vi "wymiennik ciepla z recyklem.vi"() -> ()   [LabVIEW 2013]
uses:
  <vilib>/Utility/file.llb/Write To Spreadsheet File (DBL).vi
panel:
  in  "Time STOP":bool=TRUE
  out "Tex deg.C":dbl=5.0
  out "F l/min":dbl=3.6999999999999997
  in  "Enable temperature profiles":bool=TRUE
  out "?":dbl[][](graph)=[[79.48766614690592, 79.44291247956771, 79.39728659693863, 79.35077150019917, 79.30334985923562, 79.25500400618341, 79.20571592884455, 79.15546726397692, 79.1042392904526, 79.05201292228297, 78.99876870150788, 78.94448679094619, 78.889146966805, 78.83272861114493, 78.77521070419847, 78.71657181653867, 78.6567901010952, 78.59584328501471, 78.53370866136277, 78.47036308066384, 78.40578294227656, 78.33994418560081, 78.27282228111352, 78.20439222122963, 78.1346285109851, 78.06350515853822, 77.99099566548585, 77.91707301699094, 77.84170967171757, 77.76487755156991, 77.68654803123121, 77.60669192749882, 77.52527948841141, 77.44228038216438, 77.35766368580904, 77.27139787373171, 77.18345080590827, 77.09378971592965, 77.00238119879418, 76.90919119846187, 76.81418499516609, 76.71732719247811, 76.61858170411948, 76.51791174051729, 76.41527979509759, 76.31064763031151, 76.20397626338914, 76.09522595181573, 75.98435617852483, 75.87132563680287, 75.75609221489948, 75.63861298033804, 75.51884416392022, 75.39674114341899, 75.2722584269537, 75.14534963604116, 75.01596748831648, 74.88406377991706, 74.7495893675233, 74.61249415004929, 74.47272704997664, 74.33023599432462, 74.18496789524929, 74.03686863026455, 73.88588302207783, 73.73195481803263, 73.57502666915053, 73.41504010876469, 73.2519355307369, 73.08565216725025, 72.91612806616875, 72.74330006795597, 72.56710378214362, 72.38747356334164, 72.20434248678075, 72.01764232337828, 71.8273035143181, 71.63325514513511, 71.43542491929466, 71.23373913125705, 71.0281226390171, 70.81849883610849, 70.60478962306254, 70.38691537831073, 70.16479492852007, 69.93834551835042, 69.70748277962235, 69.47212069988414, 69.23217159036608, 68.98754605331037, 68.7381529486642, 68.4838993601237, 68.22469056051622, 67.9604299765078, 67.69101915262286, 67.41635771456275, 67.13634333180926, 66.85087167949942, 66.5598363995572, 66.26312906106772, 65.96063911987918], [71.36651285431357, 71.1634840219988, 70.95649831055961, 70.74547860340017, 70.53034628098024, 70.31102119152389, 70.08742162115745, 69.8594642634653, 69.62706418845255, 69.39013481090258, 69.1485878581181, 68.9023333370334, 68.65127950068562, 68.39533281403267, 68.1343979191049, 67.8683775994776, 67.59717274405111, 67.32068231012504, 67.03880328575283, 66.75143065136263, 66.45845734063013, 66.15977420058901, 65.85526995096376, 65.54483114271005, 65.2283421157471, 64.90568495586618, 64.57673945079941, 64.24138304543229, 63.89949079614336, 63.55093532425402, 63.19558676857114, 62.833312737004654, 62.46397825724232, 62.08744572646311, 61.703574860070596, 61.312222639427155, 60.91324325856956, 60.50648806988611, 60.09180552873504, 59.66904113698357, 59.23803738544663, 58.79863369520366, 58.35066635777182, 57.893968474113144, 57.428369892453055, 56.95369714488696, 56.46977338275136, 55.97641831073543, 55.47344811970844, 54.960675418238054, 54.43790916277395, 53.90495458647083, 53.361613126624164, 52.80768235069178, 52.242955880873616, 51.667223317221634, 51.080270159251164, 50.48187772602455, 49.87182307467725, 49.24987891735612, 48.61581353653881, 47.96939069870288, 47.31036956631235, 46.638504608088944, 45.95354550753457, 45.255237069671004, 44.54331912596198, 43.817526437382284, 43.07758859559774, 42.32322992221928, 41.55416936609352, 40.77012039859166, 39.970790906857566, 39.15588308497543, 38.32509332301629, 37.4781120939222, 36.614623838185814, 35.73430684628252, 34.83683313881122, 33.921868344299156, 32.98907157462523, 32.03809529801545, 31.06858520956314, 30.08018009922566, 29.072511717248542, 28.045204636966762, 26.99787611493218, 25.930135948314934, 24.84158632952571, 23.73182169800471, 22.600428589122075, 21.44698548013353, 20.271062633133784, 19.07222193494923, 17.850016733910273, 16.603991673442465, 15.333682522414465, 14.038616002179598, 12.718309610246605, 11.372271440513844, 10.0]]
  in  "Ph":dbl(knob)=1.0 caption="C %" min=0.0 max=1.0 step=0.001 scale=0.0..1.0
  in  "Automation mode":u8(knob)=2 caption="C %" scale=0.0..2.0
  out "Ph":dbl(knob)=1.0 scale=0.0..1.0
  out "F l/min":dbl(knob)=3.6999999999999997 scale=0.0..5.0
  out "Fc l/min":dbl(knob)=0.7999999999999993 scale=0.0..5.0
  in  "?":bool
  in  "?":bool
  out "Txou deg. C":dbl=65.96063911987918
  out "Txin deg.C":dbl=79.48766614690592
  out "Tcou deg.C":dbl=71.36651285431357
  out "Fc l/min":dbl=0.7999999999999993
  out "Tcin deg.C":dbl=10.0
  in  "Auto":bool
  in  "Scaled RT interval":dbl min=0.001 max=2.0 step=0.001 format="%.3f"
  in  "NIS":dbl=600.0 min=0.0 step=1.0
  in  "Dt":dbl=1.0 min=0.0 step=1.0
  out "t  min\nmin]":dbl=2484.1883333711858
  in  "Tab Control":enum32{"Parameters ", "Manual", "Auto"}(tab)
  in  "Vh [l]":dbl=0.25 min=0.0 step=0.01 format="%.2f"
  in  "Vc [l]":dbl=0.8 min=0.0 step=0.1 format="%.1f"
  in  "Vx [l]":dbl=0.8 min=0.0 step=0.1 format="%.1f"
  in  "n":u32=100 min=2 step=1
  in  "hc[l/min]":dbl=2.0 min=0.0 step=1.0 format="%.2f"
  in  "hx[l/min]":dbl=2.0 min=0.0 step=1.0 format="%.2f"
  in  "ah [deg.C*l/min]":dbl=50.05 min=0.0 step=1.0 format="%.1f"
  in  "bc [l/min]":dbl min=0.0 step=0.05 format="%.2f"
  in  "bx[l/min]":dbl min=0.0 step=0.05 format="%.2f"
  in  "bh[l/min]":dbl min=0.0 step=0.05 format="%.2f"
  in  "Tcin [deg.C]":dbl=10.0 min=0.0 step=1.0
  in  "Fc [l/min]":dbl=0.7999999999999993 min=0.0 step=0.1 format="%.1f"
  in  "F [l/min]":dbl=3.6999999999999997 min=0.0 step=0.1 format="%.1f"
  in  "Thin [deg.C]":dbl=10.0 min=0.0 step=1.0
  in  "Tex[deg.C]":dbl=5.0 min=0.0 step=1.0
  in  "Fcmax [l/min]":dbl=4.0 min=0.0 step=0.1 format="%.1f"
  in  "Fmax [l/min]":dbl=4.0 min=0.0 step=0.1 format="%.1f"
  in  "Fcmin [l/min]":dbl=0.8 min=0.0 step=0.1 format="%.1f"
  in  "Steady state [min]":dbl=10.0 min=0.0 step=1.0
  in  "N2":dbl=10.0 min=0.0 step=1.0
  in  "Phmin":dbl=0.5 min=0.0 step=0.1 format="%.1f"
  in  "Fmin [l/min]":dbl=0.8 min=0.0 step=0.1 format="%.1f"
  in  "Phmax":dbl=1.0 min=0.0 max=1.0 step=0.1 format="%.1f"
  in  "N1":dbl=10.0 min=0.0 step=1.0
  out "Time charts":T1(graph)={"Tkoncowa"=71.36651285431357, "F2auto"=79.48766614690592, 65.96063911987918, "F1auto"=3.6999999999999997, "Twy"=0.7999999999999993, "Twe"=1.0}
  # "Tcou"
  # "80"
  # "deg.C"
  # "10"
  # "Txin/Thou"
  # "90"
  # "deg.C"
  # "10"
  # "Txou/Thin"
  # "50"
  # "deg.C"
  # "10"
  # "F"
  # "5"
  # "l/min"
  # "0"
  # "Fc"
  # "5"
  # "l/min"
  # "Manual"
  # "0"
  # "Ph"
  # "1"
  # "0"
  # "Fc"
  # "F"
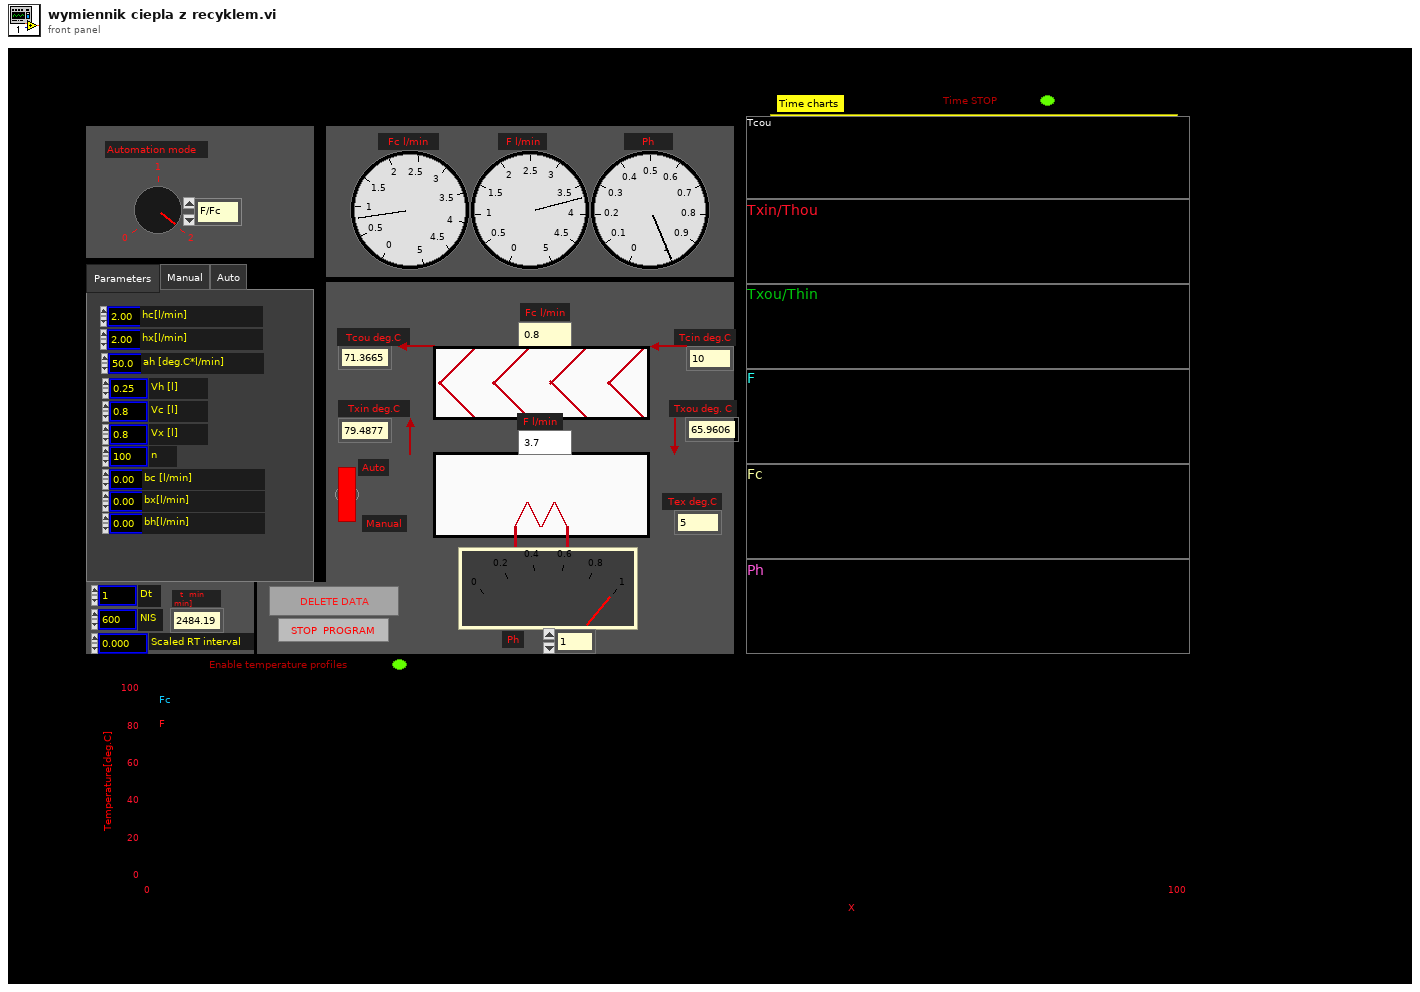
[diagram p1: front panel]
types:
  T1 = cluster{"Tkoncowa":dbl, "F2auto":dbl, dbl, "F1auto":dbl, "Twy":dbl, "Twe":dbl}
  T2 = cluster{"Tkoncowa":dbl, "Twy":dbl, "Twe":dbl, dbl, dbl, dbl}
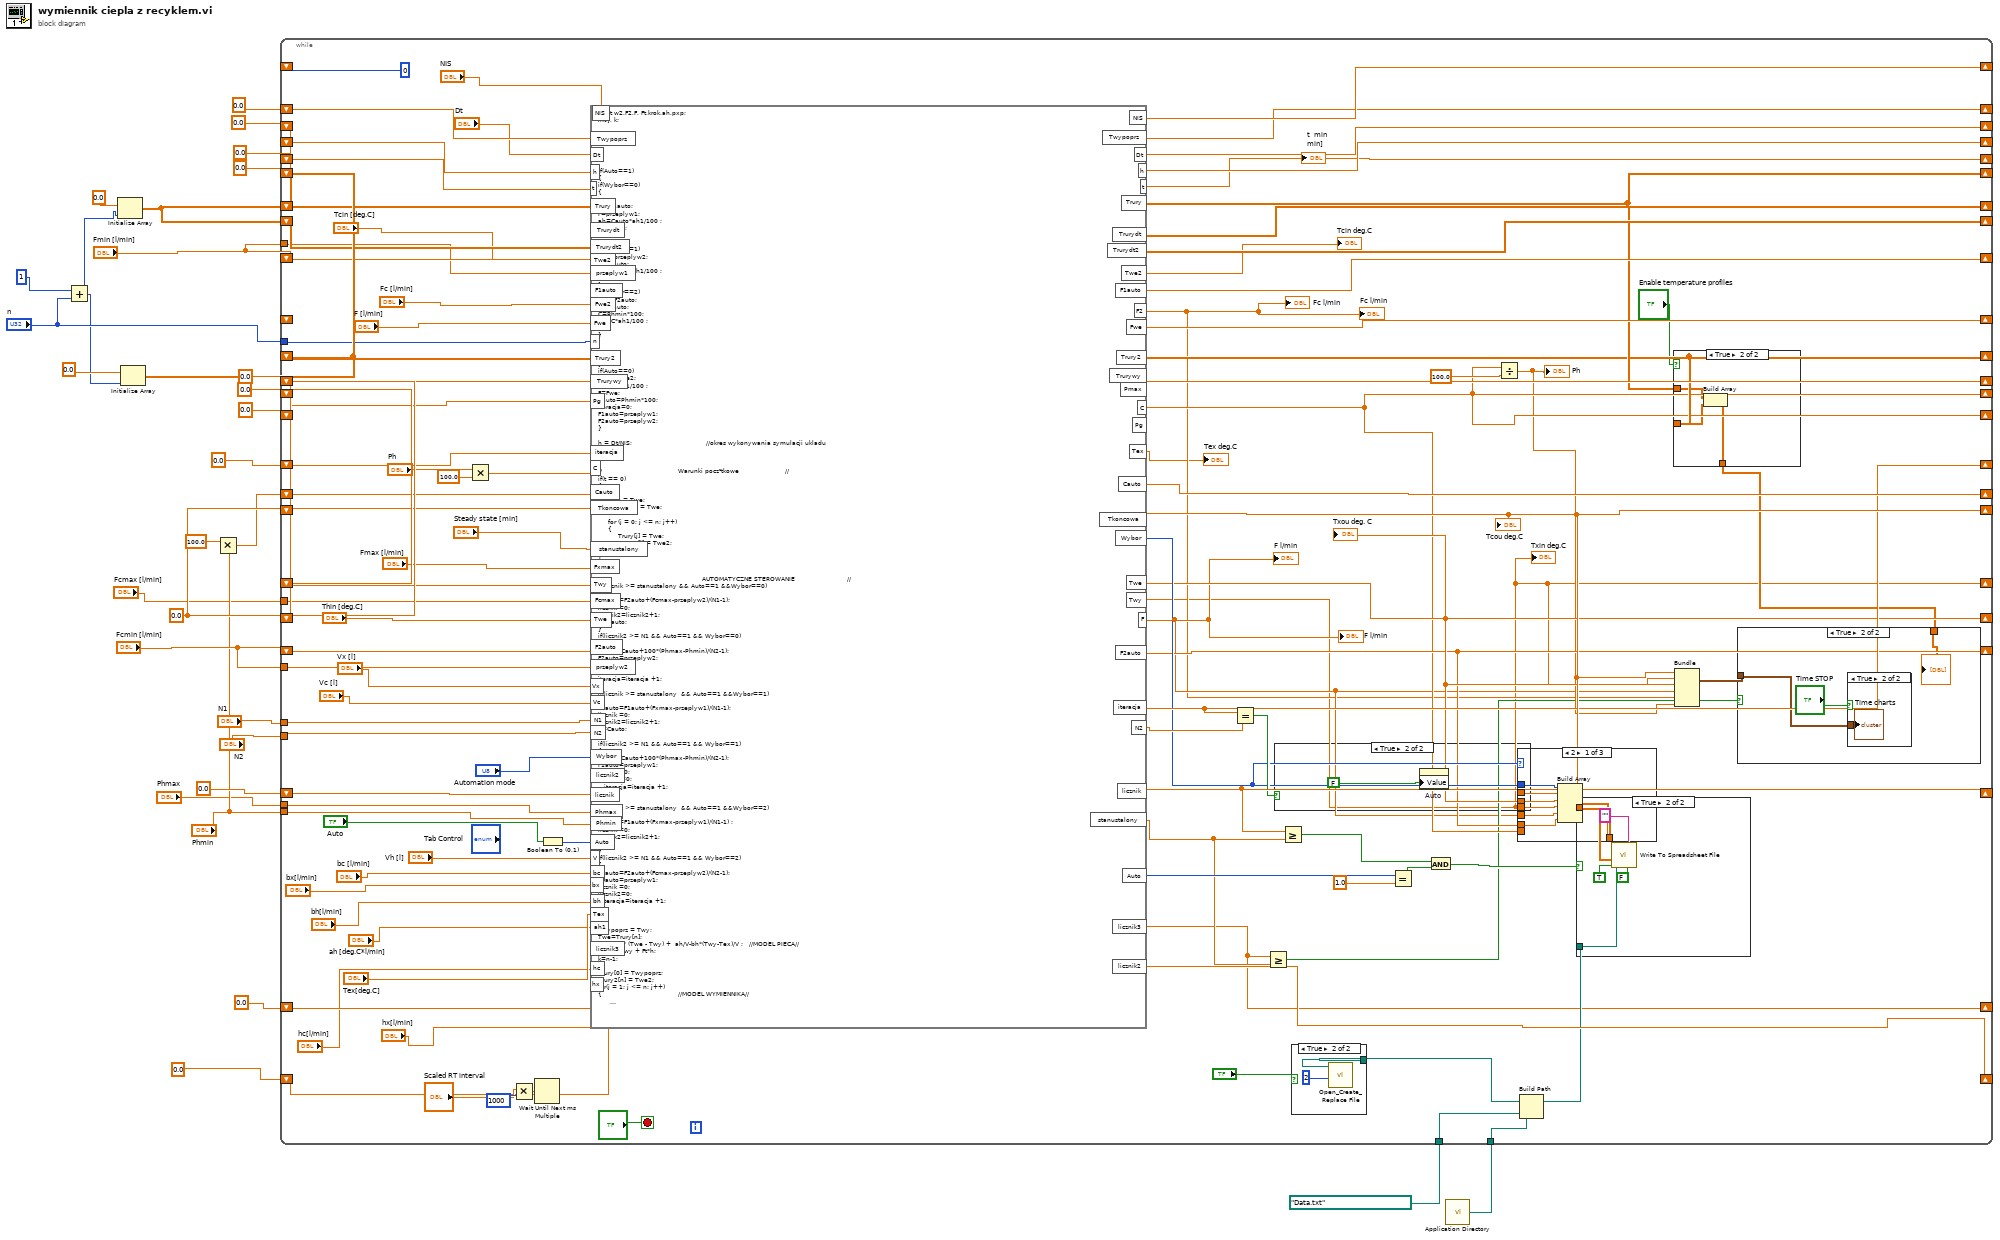
[diagram p0: block diagram]
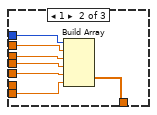
[diagram p5: hidden frame]
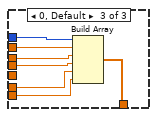
[diagram p6: hidden frame]
diagram:
  w19 = 0.0
  n1 = Add(x=1, y="n") -> (x+y=w2:u32)
  n2 = Initialize Array "Initialize Array"(0.0, w2) -> (w21:dbl[])
  n3 = Initialize Array "Initialize Array"(0.0, w2) -> (w22:dbl[])
  n4 = Multiply(x=100.0, y="Phmin") -> (x*y=w9:dbl)
  n5 = call <vilib>:"Application Directory.vi"() -> ("Application Directory"=w16:path)
  n6 = while {
    shift-right: [w106] -> _
    shift-left: 0.0 -> [w115]
    shift-right: [w32] -> _
    shift-left: 0.0 -> [w131]
    shift-right: [w110] -> _
    shift-left: 0.0 -> [w130]
    shift-right: [w122] -> _
    shift-left: 0.0 -> [w129]
    shift-right: [w52] -> _
    shift-left: _ -> [_]
    shift-right: [w77] -> _
    shift-left: 0.0 -> [_]
    shift-right: [w60] -> _
    shift-left: w22 -> [w128]
    shift-right: [w120] -> _
    shift-left: w21 -> [w119]
    shift-right: [w89] -> _
    shift-left: w19 -> [w127]
    shift-right: [w121] -> _
    shift-left: 0 -> [_]
    shift-right: [w123] -> _
    shift-left: 0.0 -> [_]
    shift-right: [w59] -> _
    shift-left: w22 -> [w118]
    shift-right: [w116] -> _
    shift-left: w21 -> [w117]
    shift-right: [w114] -> _
    shift-left: _ -> [_]
    shift-right: [w75] -> _
    shift-left: "Fcmin [l/min]" -> [w113]
    shift-right: [w111] -> _
    shift-left: 0.0 ("licznik") -> [w112]
    shift-right: [w88] -> _
    shift-left: 0.0 ("licznik") -> [w57]
    shift-right: [w86] -> _
    shift-left: w19 -> [w109]
    shift-right: [w87] -> _
    shift-left: w9 -> [w101]
    shift-right: [w52] -> _
    shift-left: 0.0 -> [w100]
    shift-right: [w76] -> _
    shift-left: "Fmin [l/min]" -> [w99]
    tunnel: "Fcmin [l/min]" -> [w97]
    tunnel: "Fmin [l/min]" -> [w96]
    shift-right: [w84] -> _
    shift-left: 0.0 ("licznik") -> [w92]
    tunnel: w16 -> [w91]
    tunnel: path "Data.txt" -> [w90]
    tunnel: "N1" -> [w83]
    tunnel: "N2" -> [w82]
    tunnel: "Phmin" -> [w64]
    tunnel: "Fcmax [l/min]" -> [w63]
    tunnel: "Phmax" -> [w62]
    tunnel: "n" -> [w61]
    shift-right: [w46] -> _
    shift-left: 0.0 ("licznik") -> [w47]
    stop <- "?" stop-if-true
    n7 = Multiply(x="Ph", y=100.0) -> (x*y=w56:dbl)
    n8 = Multiply(x="Scaled RT interval", y=1000) -> (x*y=w124:dbl)
    n9 = Wait Until Next ms Multiple(millisecond multiple=w124) -> ()  [unwired: 1 out]
    n10 = Boolean To (0,1)(Boolean="Auto") -> (0, 1=w108:i16)
    n11 = formula code="float w2,F2,F, Ft,krok,ah,pxp;\nint j, k;\n\n\n\n\n\n\nif(Auto==1) \n{\nif(Wybor==0) \n{\n\nF2=F2auto;\nF=przeplyw1;\nah=Cauto*ah1/100 ;\nC=Cauto;\n}\nF=F1auto;\nif(Wybor==1) \n{F2=przeplyw2;\nF=F1auto;\nah=Cauto*ah1/100 ;\nC=Cauto;\n}\nif(Wybor==2) \n{F2=F2auto;\nF=F1auto;\nC=Phmin*100;\nah=C*ah1/100 ;   \n\n}\n\n\n\n}\nif(Auto==0) \n{F2 = Fwe2; \nah=C*ah1/100 ;     \nF=Fwe;\nCauto=Phmin*100;\niteracja=0;\nF1auto=przeplyw1;\nF2auto=przeplyw2;\n}\n\nh = Dt/NIS;                                     //okres wykonywania symulacji ukladu                                       \n\n\n\n//                                      Warunki pocz¹tkowe                       //\nif(t == 0)\n{\n \n     Twy = Twe;\n     Twypoprz = Twe;\n\n     for (j = 0; j <= n; j++)\n     {\n          Trury[j] = Twe;\n          Trury2[j] = Twe2;\n     }\n}\n\n\n//                                                  AUTOMATYCZNE STEROWANIE                          //\nif(licznik >= stanustalony && Auto==1 &&Wybor==0) \n{\nF2auto=F2auto+(Fcmax-przeplyw2)/(N1-1);\nlicznik =0;\nlicznik2=licznik2+1;\nC=Cauto;\n}\nif(licznik2 >= N1 && Auto==1 && Wybor==0)\n{\nCauto=Cauto+100*(Phmax-Phmin)/(N2-1);\nF2auto=przeplyw2;\nlicznik =0;\nlicznik2=0;\niteracja=iteracja +1;\n}\nif(licznik >= stanustalony  && Auto==1 &&Wybor==1) \n{\nF1auto=F1auto+(Fxmax-przeplyw1)/(N1-1);\nlicznik =0;\nlicznik2=licznik2+1;\nC=Cauto;\n}\nif(licznik2 >= N1 && Auto==1 && Wybor==1)\n{\nCauto=Cauto+100*(Phmax-Phmin)/(N2-1);\nF1auto=przeplyw1;\nlicznik =0;\nlicznik2=0;\n   iteracja=iteracja +1;\n}\n\nif(licznik >= stanustalony  && Auto==1 &&Wybor==2) \n{\nF1auto=F1auto+(Fxmax-przeplyw1)/(N1-1) ;\nlicznik =0;\nlicznik2=licznik2+1;\n\n}\nif(licznik2 >= N1 && Auto==1 && Wybor==2)\n{\nF2auto=F2auto+(Fcmax-przeplyw2)/(N2-1);\nF1auto=przeplyw1;\nlicznik =0;\nlicznik2=0;\n  iteracja=iteracja +1; \n}\n\n\nTwypoprz = Twy;\nTwe=Trury[n];         \nFt = F/V * (Twe - Twy) +  ah/V-bh*(Twy-Tex)/V ;   //MODEL PIECA//\nTwy = Twy + Ft*h; \nk=n-1;\n\nTrury[0] = Twypoprz;\nTrury2[n] = Twe2;\nfor(j = 1; j <= n; j++)\n{                                      //MODEL WYMIENNIKA//\n      Trurydt[j] = n*F*(Trury[j-1] - Trury[j])/Vx - hx * (Trury[j] -  Trury2[j])/Vx - bx*(Trury[j] -  Tex)/Vx;                      \n     Trurydt2[k] =n*F2* (Trury2[k+1] - Trury2[k])/Vc +hc* (Trury[k] -  Trury2[k])/Vc- bc*(Trury2[k] -  Tex)/Vc;   \n\n      k=k-1;\n}\nk=n-1;\nfor(j = 1; j <= n; j++)\n{\n     Trury[j] = Trury[j] + Trurydt[j]*h;\n     Trury2[k] = Trury2[k] + Trurydt2[k]*h;\n      k=k-1;\n}\nTkoncowa=Trury2[0] ;\nif(Auto==1)\n{licznik=licznik+h;\n}\nt = t + h;\nlicznik3=licznik3+h;\nif(licznik3>stanustalony+h)\n{licznik3=0;\n}"("t"=w115, "Fwe"="F [l/min]", "Twe"="Thin [deg.C]", "C"=w56, "Trurydt"=w119, "Trury"=w128, "Twy"=w131, "Twypoprz"=w130, "NIS"="NIS", "Dt"="Dt", "h"=w129, "Trurywy"=w127, "Trury2"=w118, "Trurydt2"=w117, "Fwe2"="Fc [l/min]", "Twe2"="Tcin [deg.C]", "V"="Vh [l]", "F2auto"=w113, "licznik"=w112, "licznik2"=w57, "Tkoncowa"=w109, "Auto"=w108, "Cauto"=w101, "Pg"=w100, "F1auto"=w99, "Wybor"="Automation mode", "przeplyw2"=w97, "przeplyw1"=w96, "iteracja"=w92, "stanustalony"="Steady state [min]", "Vx"="Vx [l]", "Vc"="Vc [l]", "Fcmax"=w63, "Fxmax"="Fmax [l/min]", "N1"=w83, "N2"=w82, "Phmax"=w62, "Phmin"=w64, "n"=w61, "hc"="hc[l/min]", "hx"="hx[l/min]", "ah1"="ah [deg.C*l/min]", "bc"="bc [l/min]", "bx"="bx[l/min]", "bh"="bh[l/min]", "Tex"="Tex[deg.C]", "licznik3"=w47) -> ("Twy"=w32:dbl, "Trury"=w60:dbl[], "Twe"=w77:dbl, "Twypoprz"=w110:dbl, "NIS"=w121:dbl, "Dt"=w123:dbl, "h"=w122:dbl, "t"=w106:dbl, "Fwe"=w114:dbl, "C"=w52:dbl, "Trurydt"=w120:dbl[], "Trurywy"=w89:dbl, "Trury2"=w59:dbl[], "Trurydt2"=w116:dbl[], "F2auto"=w75:dbl, "licznik"=w111:dbl, "licznik2"=w88:dbl, "Cauto"=w87:dbl, "Tkoncowa"=w86:dbl, "Twe2"=→"Tcin deg.C":dbl, "F2"=w42:dbl, "Auto"=w103:i16, "F1auto"=w76:dbl, "F"=w43:dbl, "Wybor"=w78:u8, "iteracja"=w84:dbl, "stanustalony"=w49:dbl, "N2"=w81:dbl, "licznik3"=w46:dbl, "Tex"=→"Tex deg.C":dbl)  [unwired: 2 out]
    "t  min\nmin]" <- w106
    "Fc l/min" <- w42
    "Tcou deg.C" <- w86
    "Txin deg.C" <- w32
    "Txou deg. C" <- w77
    "F l/min" <- w43
    "Fc l/min" <- w42
    "F l/min" <- w43
    n12 = Equal?(x=w84, y=w81) -> (x = y?=w85:bool)
    n13 = Greater Or Equal?(x=w46, y=w49) -> (x >= y?=w48:bool)
    n14 = case shown="True" w85 {
      frame False {
      }
      frame True {
        n15 = property on="Auto" class="Bool (strict)"("Value"=FALSE) -> ()  [unwired: 2 in, 2 out]
      }
    }
    n16 = Greater Or Equal?(x=w111, y=w49) -> (x >= y?=w105:bool)
    n17 = Equal?(x=w103, y=1.0) -> (x = y?=w102:bool)
    n18 = And(x=w105, y=w102) -> (x .and. y?=w95:bool)
    n19 = Divide(x=w52, y=100.0) -> (x/y=w51:dbl)
    "Ph" <- w51
    n20 = case shown="2" w78 {
      tunnel: w77 -> [w142 w147 w156]
      tunnel: w43 -> [w140 w151 _]
      tunnel: w78 -> [w144 w149 w159]
      tunnel: [w145 w152 w158] -> w93
      tunnel: w32 -> [w141 w146 w155]
      tunnel: w75 -> [w139 _ w154]
      tunnel: w52 -> [_ w150 w153]
      tunnel: w86 -> [w143 w148 w157]
      frame 2 {
        n21 = Build Array(w144, w143, w142, w141, w140, w139) -> (w145:dbl[])
      }
      frame 1 {
        n22 = Build Array(w149, w148, w147, w146, w151, w150) -> (w152:dbl[])
      }
      frame 0, Default {
        n23 = Build Array(w159, w157, w156, w155, w154, w153) -> (w158:dbl[])
      }
    }
    n24 = Build Path(base path=w91, name or relative path=w90) -> (appended path=w79:path)
    n25 = case shown="True" "?" {
      tunnel: w79 -> [_ w160]
      frame False {
      }
      frame True {
        n26 = call <vilib>:"Open_Create_Replace File.vi"("function (open:0)"=2, "file path"=w160) -> ()  [unwired: 6 in, 4 out]
      }
    }
    n27 = case shown="True" w95 {
      tunnel: w93 -> [_ w162]
      tunnel: w79 -> [_ w164]
      frame False {
      }
      frame True {
        n28 = call-poly <vilib>:"Write To Spreadsheet File.vi"("transpose? (no:F)"=FALSE, "format (%.3f)"="", "append to file? (new file:F)"=TRUE, "1D data"=w162, "file path (dialog if empty)"=w164) -> ()  [unwired: 3 in, 1 out]
      }
    }
    n29 = case shown="True" "Enable temperature profiles" {
      tunnel: w60 -> [_ w138]
      tunnel: w59 -> [_ w137]
      tunnel: [_ w136] -> w45
      frame False {
      }
      frame True {
        n30 = Build Array(w138, w137) -> (w136:dbl[][])
      }
    }
    n31 = Bundle("Tkoncowa"=w86, "Twy"=w32, "Twe"=w77, w43, w42, w51) -> (w44:T2)  [unwired: 1 in]
    n32 = case shown="True" w48 {
      tunnel: w45 -> [_ w134]
      tunnel: w44 -> [_ w133]
      frame False {
      }
      frame True {
        n33 = case shown="True" "Time STOP" {
          tunnel: w133 -> [_ w135]
          frame False {
          }
          frame True {
            "Time charts" <- w135
          }
        }
        "?" <- w134
      }
    }
  }
